vi "Simulate IM Measurement.vi"(5 "Measurement Results In":T9 {"IMPower_dBc(s)" format="%.2f"; "TxFreqs" format="%.2f"; "IMFreq(s)" format="%.2f"; "IMPower(s)" format="%.2f"; "TxPower" format="%.2f"}, 8 "Simulate Response Lag (50ms)":u32=50, 9 "Average IM (-120 dBm)":dbl=-120.0, 10 "Low-side?":bool, 11 "Stimulus":T1 {"Measurement Setup"."TXStep" items=[".2", ".4", "1.0", "2.0"]; "Measurement Parameters"."Direction" items=["Reverse", "Forward", "Auxiliary"]; "Measurement Parameters"."IM Order" items=["3rd", "5th", "7th", "9th", "11th", "13th", "15th", "17th", "19th", "21st", "23rd", "25th", "27th", "29th", "31st", "33rd"]; "Measurement Parameters"."Averaging" items=["None", "Minimum", "Normal", "High", "Maximum"]}) -> (3 "Measurement Results Out":T9 {"IMPower_dBc(s)" format="%.2f"; "TxFreqs" format="%.2f"; "IMFreq(s)" format="%.2f"; "IMPower(s)" format="%.2f"; "TxPower" format="%.2f"})   [LabVIEW 2011]
uses:
  PIM Results.ctl
  PIM Stimulus.ctl
  PIM Cmd Params.ctl
  SI.LIB/PIM.LIB/HW IO/IMOrder.ctl
  SI.LIB/PIM.LIB/HW IO/HW Averaging.ctl
  SI.LIB/PIM.LIB/HW IO/MeasMode.ctl
  SI.LIB/PIM.LIB/DISPLAY/display_unit_format.ctl
  SI.LIB/PIM.LIB/HW IO/DUTport.ctl
  SI.LIB/PIM.LIB/HW IO/PIM Sweep Step Size.ctl
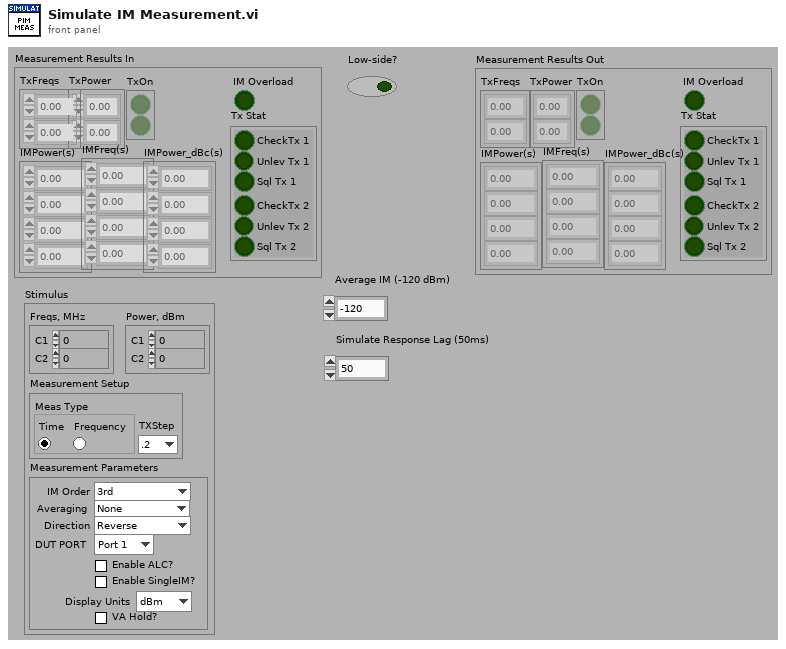
[diagram p1: front panel]
types:
  T1 = typedef "PIM Stimulus.ctl" = cluster{"Carrier Frequencies":cluster{"C1 Freq, MHz":dbl, "C2 Freq, MHz":dbl}, "Carrier Powers":cluster{"C1 Power,dBm":dbl, "C2 Power, dBm":dbl}, "Measurement Parameters":T2, "Measurement Setup":cluster{"Meas Type":enum32{"Time", "Frequency"}, "TXStep":T8}}
  T2 = typedef "PIM Cmd Params.ctl" = cluster{"IM Order":T3, "Averaging":T4, "Direction":T5, "Enable ALC?":bool, "Enable SingleIM?":bool, "Display Units":T6, "VA Hold?":bool, "DUT PORT":T7}
  T3 = typedef "IMOrder.ctl" = u8
  T4 = typedef "HW Averaging.ctl" = u16
  T5 = typedef "MeasMode.ctl" = u16
  T6 = typedef "display_unit_format.ctl" = enum16{"dBm", "dBc"}
  T7 = typedef "DUTport.ctl" = enum16{"Port 1", "Port 2"}
  T8 = typedef "PIM Sweep Step Size.ctl" = u16
  T9 = typedef "PIM Results.ctl" = cluster{"TxFreqs":dbl[], "TxPower":dbl[], "TxOn":bool[], "IMPower(s)":dbl[], "IMFreq(s)":dbl[], "Tx Stat":cluster{"CheckTx 1":bool, "Unlev Tx 1":bool, "Sql Tx 1":bool, "CheckTx 2":bool, "Unlev Tx 2":bool, "Sql Tx 2":bool}, "IM Overload":bool, "IMPower_dBc(s)":dbl[]}
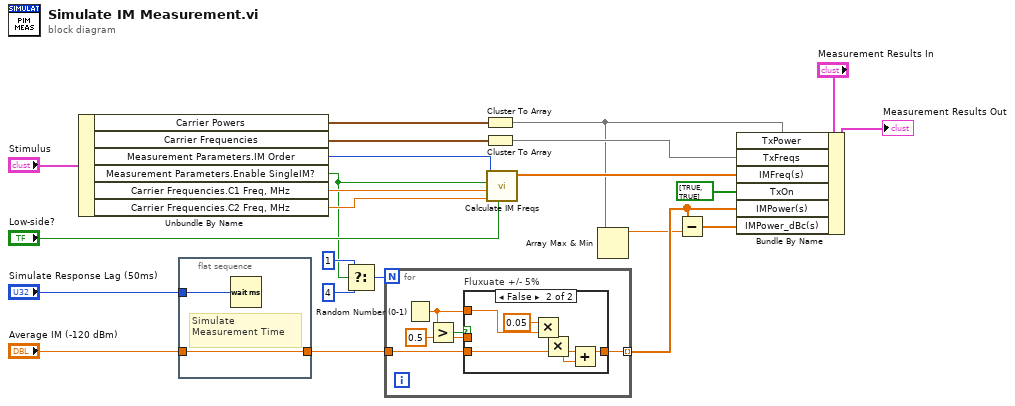
[diagram p0: block diagram]
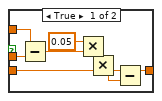
[diagram p2: hidden frame]
diagram:
  n1 = Unbundle By Name("Stimulus") -> ("Carrier Powers"=w15:cluster{"C1 Power,dBm":dbl, "C2 Power, dBm":dbl}, "Carrier Frequencies"=w14:cluster{"C1 Freq, MHz":dbl, "C2 Freq, MHz":dbl}, "Measurement Parameters.IM Order"=w19:T3, "Measurement Parameters.Enable SingleIM?"=w9:bool, "Carrier Frequencies.C1 Freq, MHz"=w17:dbl, "Carrier Frequencies.C2 Freq, MHz"=w18:dbl)
  n2 = flat-sequence {
    tunnel: "Simulate Response Lag (50ms)" -> [w25]
    tunnel: "Average IM (-120 dBm)" -> [w24]
    tunnel: [w24] -> w1
    frame #0 {
      # "Simulate Measurement Time"
      n3 = Wait (ms)(milliseconds to wait=w25) -> ()  [unwired: 1 out]
    }
  }
  n4 = Select(t=1, s=w9, f=4) -> (s? t:f=w8:i32)
  n5 = for {
    N: w8 -> [_]
    tunnel: w1 -> [w27]
    tunnel: [w26] -> w6 mode=indexing
    w28 = 0.5 ("y")
    n6 = Random Number (0-1)() -> (number: 0 to 1=w29:dbl)
    n7 = Greater?(x=w29, y=w28) -> (0:w30:bool)
    n8 = case "Fluxuate +/- 5%" shown="False" w30 {
      tunnel: w27 -> [w33 w42]
      tunnel: w29 -> [w38 w39]
      tunnel: w28 -> [w37 _]
      tunnel: [w31 w40] -> w26
      frame True {
        n9 = Subtract(x=w38, y=w37) -> (x-y=w36:dbl)
        n10 = Multiply(x=0.05, y=w36) -> (x*y=w34:dbl)
        n11 = Multiply(x=w34, y=w33) -> (x*y=w32:dbl)
        n12 = Subtract(x=w33, y=w32) -> (x-y=w31:dbl)
      }
      frame False {
        n13 = Multiply(x=0.05, y=w39) -> (x*y=w43:dbl)
        n14 = Multiply(x=w43, y=w42) -> (x*y=w41:dbl)
        n15 = Add(x=w42, y=w41) -> (x+y=w40:dbl)
      }
    }
  }
  n16 = Cluster To Array(cluster=w15) -> (array=w7:dbl[])
  n17 = Cluster To Array(cluster=w14) -> (array=w13:dbl[])
  n18 = call "Calculate IM Freqs.vi"("Low-side?"="Low-side?", "F2 (Carrier 2)"=w18, "F1 (Carrier 1)"=w17, "SingleIM? (f)"=w9, "BaseOrder"=w19) -> ("IM Frequencies"=w22:dbl[])  [unwired: 6 in]
  n19 = Array Max & Min(array=w7) -> (max value=w5:dbl)  [unwired: 3 out]
  n20 = Subtract(x=w6, y=w5) -> (x-y=w4:dbl[])
  n21 = Bundle By Name(cluster="Measurement Results In", "TxPower"=w7, "TxFreqs"=w13, "IMFreq(s)"=w22, "TxOn"=bool[] [TRUE, TRUE], "IMPower(s)"=w6, "IMPower_dBc(s)"=w4) -> (→"Measurement Results Out":T9)
